vi "Create and Add Instrument.vi"(6 "Physical Intr Configs":string[](array[string]), 8 "Error In":errorcluster, 11 "reference in":refnum<class "Measure and Stimulus Subsystems.lvclass">) -> (0 "Error Out":errorcluster, 3 "reference out":refnum<class "Measure and Stimulus Subsystems.lvclass">)   [LabVIEW 2023, in "HAL GOOP4.lvlib" / "Measure and Stimulus Subsystems.lvclass"]
uses:
  Measure and Stimulus Subsystems.lvclass
  Measure and Stimulus Subsystems.lvclass/Measure and Stimulus Subsystems.ctl
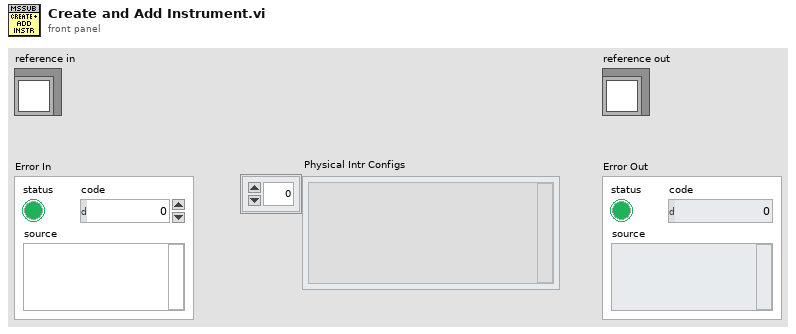
[diagram p1: front panel]
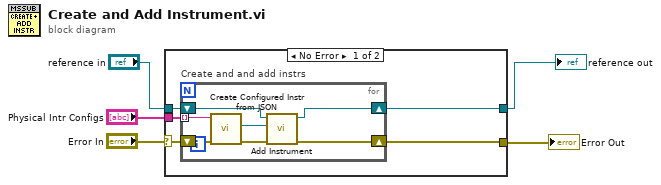
[diagram p0: block diagram]
diagram:
  n1 = case shown="No Error" "Error In" {
    selector: "Error In" -> [w7 w18]
    tunnel: [w8 w18] -> w5
    tunnel: [w9 w19] -> w4
    tunnel: "reference in" -> [w10 w19]
    tunnel: "Physical Intr Configs" -> [w6 _]
    frame No Error {
      n2 = for "Create and and add instrs" {
        shift-right: [w11] -> w8
        shift-left: w7 -> [w17]
        tunnel: w6 -> [w16] mode=indexing
        shift-right: [w12] -> w9
        shift-left: w10 -> [w13]
        n3 = call "Create Configured Instr from JSON.vi"("error in (no error)"=w17, "<JSON CFG>"=w16) -> ("error out"=w15:errorcluster, "IInstrument Base"=w14:refnum<class "Instrument.lvclass">)  [unwired: 8 in]
        n4 = call "Add Instrument.vi"("error in (no error)"=w15, "Instrument"=w14, "Measure and Stimulus Subsystems in"=w13) -> ("error out"=w11:errorcluster, "Measure and Stimulus Subsystems out"=w12:refnum<class "Measure and Stimulus Subsystems.lvclass">)  [unwired: 7 in]
      }
    }
    frame Error {
    }
  }
  "Error Out" <- w5
  "reference out" <- w4
